vi "Job.vi"(8 "error in (no error)":errorcluster) -> (0 "error out":errorcluster, 3 "VGS_Job out":refnum<class "VGS_Job.lvclass">)   [LabVIEW 2022 SP3, in "LV_VGS.lvlib" / "VGS_Job.lvclass"]
uses:
  VGS_Job.lvclass
  VGS_Job.lvclass/VGS_Job.ctl
  C:/Users/Andrey/Desktop/hajo/LV_VGS/vgs_project.dll
  vgs_project.dll
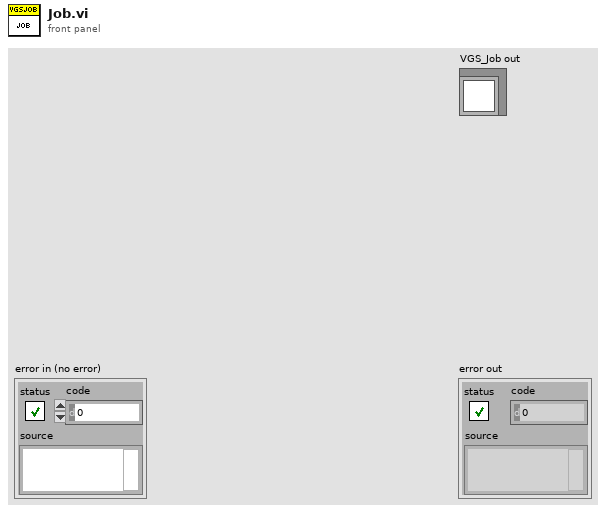
[diagram p1: front panel]
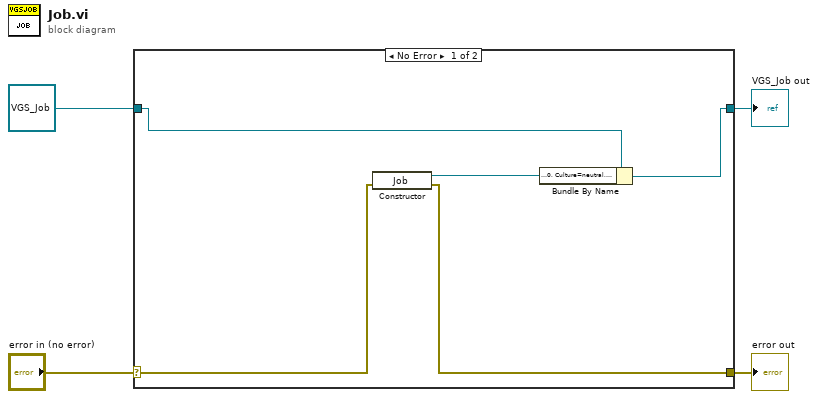
[diagram p0: block diagram]
diagram:
  n1 = case shown="No Error" "error in (no error)" {
    selector: "error in (no error)" -> [w7 w11]
    tunnel: [w6 w11] -> w3
    tunnel: [w8 w10] -> w2
    tunnel: refnum<class "VGS_Job.lvclass"> refnum ("VGS_Job in") -> [w5 w10]
    frame No Error {
      n2 = constructor class="Job"(error in=w7) -> (reference out=w9:refnum<k24>, error out=w6:errorcluster)  [unwired: 2 in, 1 out]
      n3 = Bundle By Name(cluster=w5, "Job reference"=w9) -> (w8:refnum<class "VGS_Job.lvclass">)
    }
    frame Error {
    }
  }
  "error out" <- w3
  "VGS_Job out" <- w2
